vi "disconnect.vi"(8 "error in (no error)":errorcluster, 11 "TCPServer in":refnum<class "TCPServer.lvclass">) -> (0 "error out":errorcluster, 3 "TCPServer out":refnum<class "TCPServer.lvclass">)   [LabVIEW 2016, in "TCPServer.lvclass"]
uses:
  TCPServer.lvclass
  C:/Users/aanania/Documents/ss_atdome/ts_labview_tcp/TCPCommunicator/TCPCommunicator.lvclass
  TCPCommunicator/TCPCommunicator.lvclass/TCPCommunicator.ctl
  TCPCommunicator/TCPCommunicator.lvclass
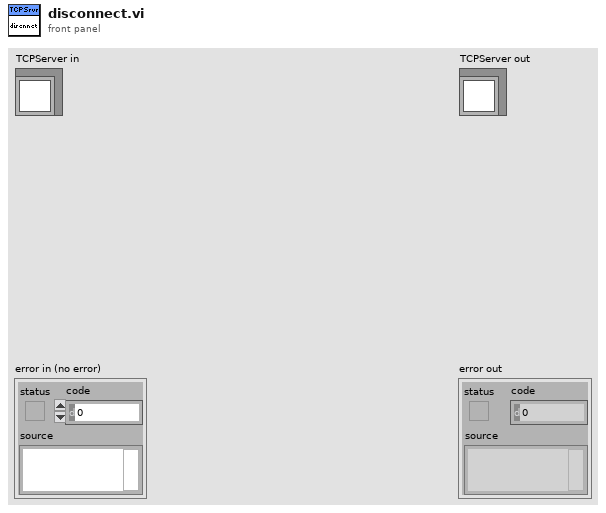
[diagram p1: front panel]
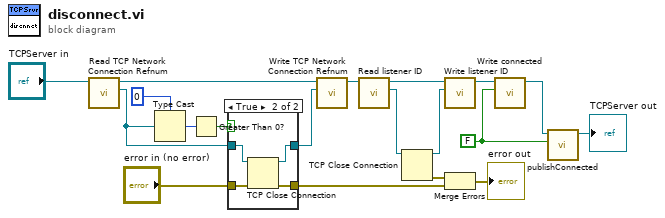
[diagram p0: block diagram]
diagram:
  w1 = FALSE ("connected")
  n1 = call-dynamic "Read TCP Network Connection Refnum.vi"("TCPCommunicator in"="TCPServer in") -> ("TCP Network Connection Refnum"=w7:refnum<k5>, "TCPCommunicator out"=w16:refnum<class "TCPServer.lvclass">)  [unwired: 8 in, 1 out]
  n2 = Type Cast(type=0, x=w7) -> (*(type *) &x=w4:i32)
  n3 = Greater Than 0?(x=w4) -> (x > 0?=w6:bool)
  n4 = case shown="True" w6 {
    tunnel: w7 -> [w20 w25]
    tunnel: "error in (no error)" -> [w21 w24]
    tunnel: [w20 w23] -> w17
    tunnel: [w21 w22] -> w10
    frame False {
    }
    frame True {
      n5 = TCP Close Connection(connection ID=w25, error in (no error)=w24) -> (connection ID out=w23:refnum<k5>, error out=w22:errorcluster)  [unwired: 1 out]
    }
  }
  n6 = call-dynamic "Write TCP Network Connection Refnum.vi"("TCP Network Connection Refnum"=w17, "TCPCommunicator in"=w16) -> ("TCPCommunicator out"=w15:refnum<class "TCPServer.lvclass">)  [unwired: 8 in, 1 out]
  n7 = call "Read listener ID.vi"("TCPCommunicator in"=w15) -> ("listener ID"=w13:refnum<k5>, "TCPCommunicator out"=w14:refnum<class "TCPServer.lvclass">)  [unwired: 8 in, 1 out]
  n8 = TCP Close Connection(connection ID=w13) -> (connection ID out=w12:refnum<k5>, error out=w9:errorcluster)  [unwired: 1 in, 1 out]
  n9 = call "Write listener ID.vi"("listener ID"=w12, "TCPCommunicator in"=w14) -> ("TCPCommunicator out"=w11:refnum<class "TCPServer.lvclass">)  [unwired: 8 in, 1 out]
  n10 = Merge Errors(w9, w10) -> (→"error out":errorcluster)
  n11 = call "Write connected.vi"("connected"=w1, "TCPCommunicator in"=w11) -> ("TCPCommunicator out"=w3:refnum<class "TCPServer.lvclass">)  [unwired: 8 in, 1 out]
  n12 = call-dynamic "publishConnected.vi"("Connected"=w1, "TCPCommunicator in"=w3) -> ("TCPCommunicator out"=→"TCPServer out":refnum<class "TCPServer.lvclass">)  [unwired: 8 in, 1 out]
